vi "RH_BF_LD-400_MFLI_PK_v4.0_measure_voltageR_fourMFLI.vi"() -> ()   [LabVIEW 2016]
uses:
  <instrlib>/Zurich Instruments LabOne/Public/Configure/ziGetValueDemodSampleEx.vi
  <vilib>/Utility/file.llb/Write To Spreadsheet File (DBL).vi
  <instrlib>/Zurich Instruments LabOne/Zurich Instruments LabOne.lvlib
panel:
  in  "Magnet IP Address":string="169.254.50.121"
  in  "Current 4 (A)":dbl
  in  "Current 3 (A)":dbl
  in  "Current 2 (A)":dbl
  in  "Current 1 (A)":dbl
  in  "MFLI 4 Address":string="DEV3647"
  in  "Device 4 details:":string="ZrTe5_Rxy_24-32_10uA_7.919Hz"
  in  "Delay(s) after each data point":dbl=8.0 format="%#_13g"
  in  "Device 3 details:":string="ZrTe5_Rxx_35-32_10uA_7.919Hz"
  in  "MFLI 3 Address":string="DEV3647"
  in  "MFLI 2 Address":string="DEV4496"
  in  "MFLI 1 Address":string="DEV4382"
  in  "Device 2 details:":string="ZrTe5_Rxx_39-24_10uA_7.919Hz"
  in  "Device 1 details:":string="ZrTe5_Rxy_39-35_10uA_7.919Hz"
  in  "STOP":bool
  out "Device details":string="Device details: \rDevice 1 details: AJ0267-Ta3Sb(21nm)/TaN(2nm)/Sapphire (RT growth)\tDevice 1 details: AJ0268-Ta3Sb(21nm)/TaN(2nm)/Sapphire (1000C growth)\r\t"
  out "data":ext[](array[numeric])=[0.0080852, 9923.583, 0.16276936015514457, 1.6064700025522405e-08, 9.869609372556507e-08, 0.27307549143227666, 2.7272832558602143e-08, 9.987286817852663e-08]
  out "path":path=path "D:/Pranava/Data/Ta3Sb/15-07-2020/001_AJ0267+AJ0268_RT_cooldown_100nA"
  in  "Path":path=path "D:/Pranava/Data/Stan/12-06-2021/002_ZrTe5_RH_baseT"
  in  "Tab Control":enum32{"Page 1", "Page 2"}(tab)
  out "Resistance vs time":cluster{dbl[], dbl[]}[](graph)
  out "Resistance 1 (ohm)":dbl=0.16276936015514457 format="%#_13g"
  out "Voltage 1 (V)":dbl=1.6064700025522405e-08 format="%#_4g"
  out "elapsed time (min)":dbl=165.39305000000002
  out "elapsed time (s)":dbl=9923.583
  out "Magnetic Field (T)":dbl=0.0080852
  out "Resistance vs T":cluster{dbl[], dbl[]}[](graph)
  out "Voltage 2 (V)":dbl=2.7272832558602143e-08 format="%#_4g"
  out "Resistance 2 (ohm)":dbl=0.27307549143227666 format="%#_13g"
  out "Resistance 3 (ohm)":dbl format="%#_13g"
  out "Voltage 3 (V)":dbl=2.7272832558602143e-08 format="%#_4g"
  out "Resistance 4 (ohm)":dbl=0.16276936015514457 format="%#_13g"
  out "Voltage 4 (V)":dbl=2.7272832558602143e-08 format="%#_4g"
  out "Updates":string="- Using shift register to get data from MFLI\n- Using read demod instead of poll function\n- Measuring 4 devices using MFLI at the same time"
  out "Error Out":errorcluster
  # "Use this button to abort the measurement"
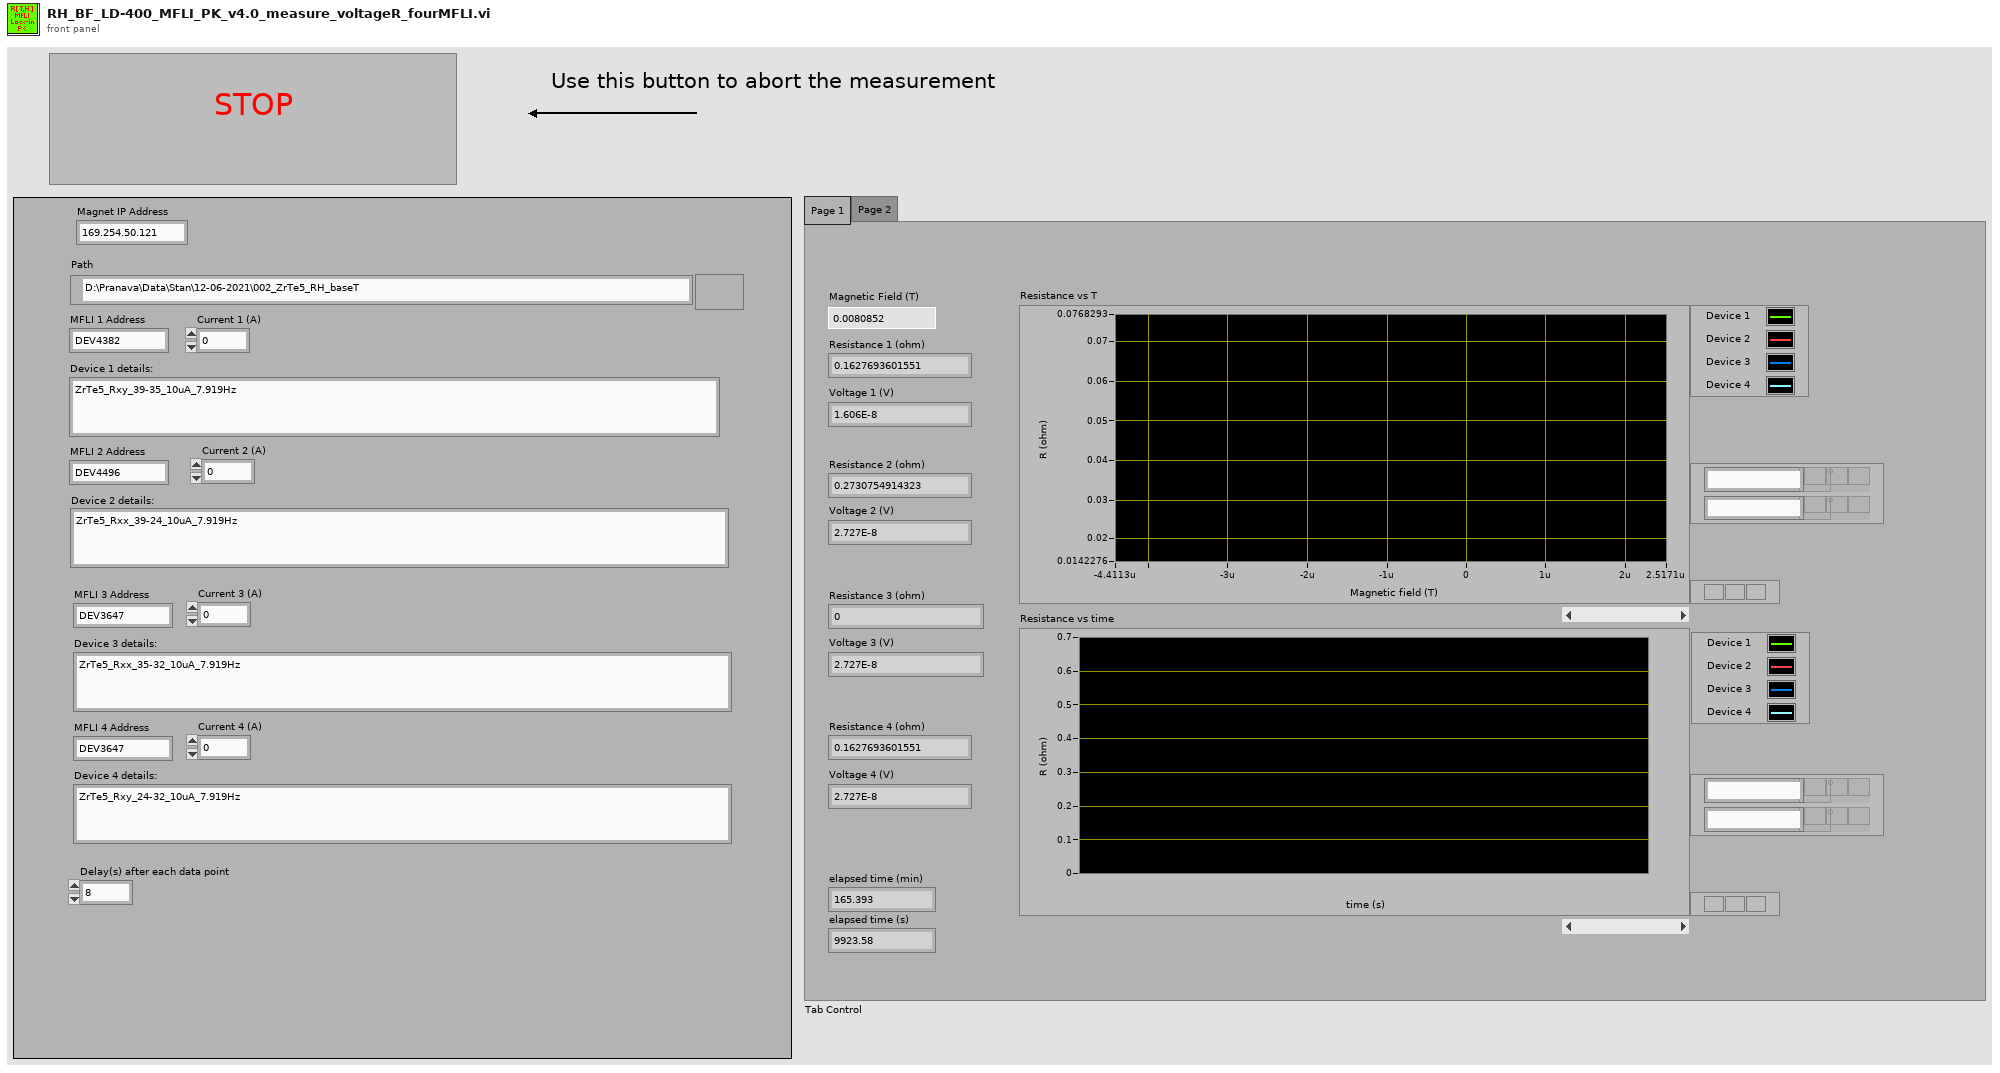
[diagram p1: front panel]
types:
  T1 = enum16{"open", "replace", "create", "open or create", "replace or create", "replace or create with confirmation"}
  T2 = typedef "Zurich Instruments LabOne.lvlib/ziTypeHandle.ctl" = cluster{"handleValid":bool, "Conn":u64, "Path Prefix":string, "Handle":u64, "Connected":bool, "Clockbase(s)":dbl}
  T3 = typedef "Zurich Instruments LabOne.lvlib/ziTypeDemodSampleSingle.ctl" = cluster{"Timestamps (ticks)":u64, "X (Vrms)":dbl, "Y (Vrms)":dbl, "Osc Phase (deg)":dbl, "Freq (Hz)":dbl, "DIO":u32, "AuxIn0 (V)":dbl, "AuxIn1 (V)":dbl, "Trigger":u32}
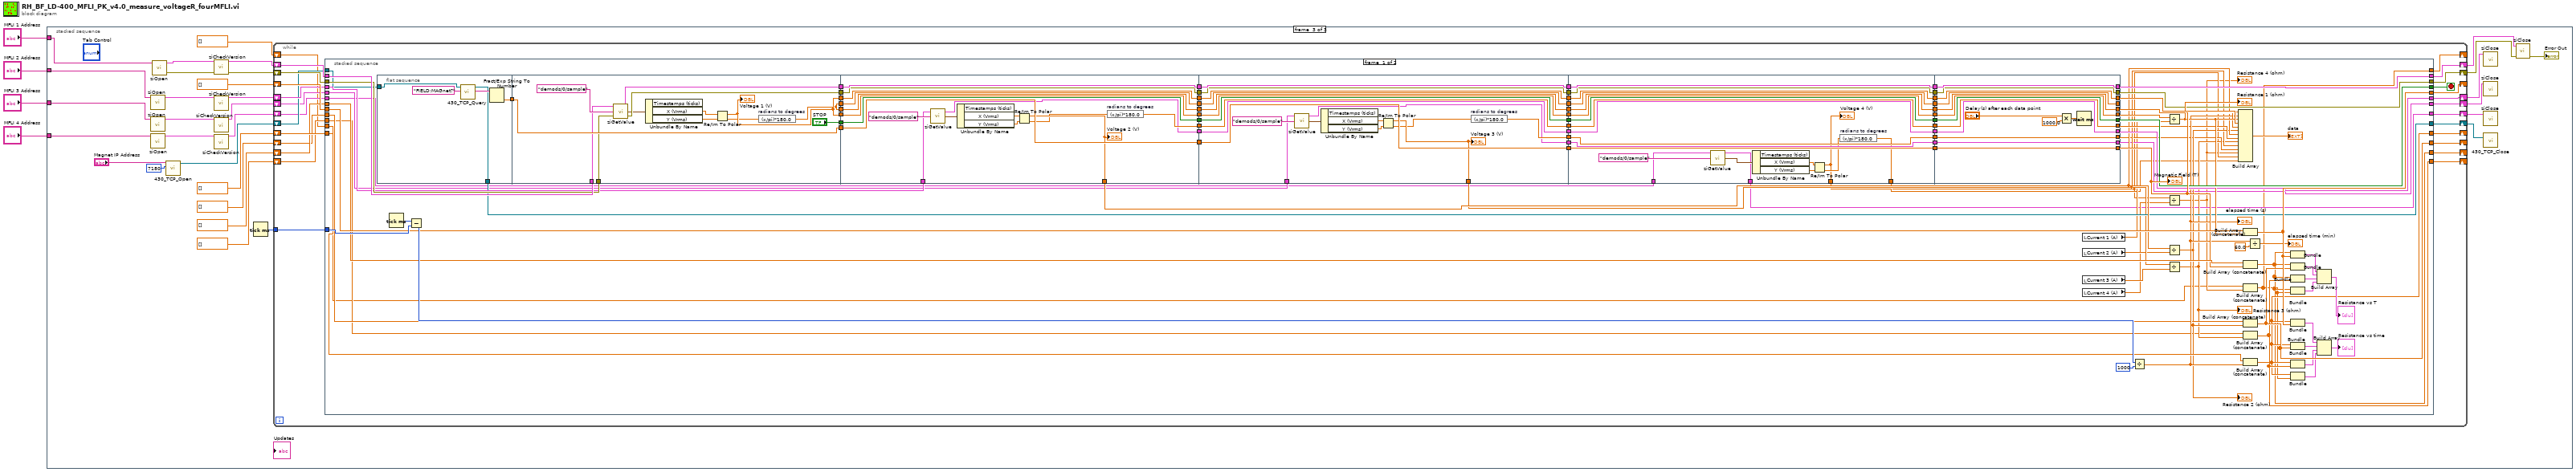
[diagram p0: block diagram]
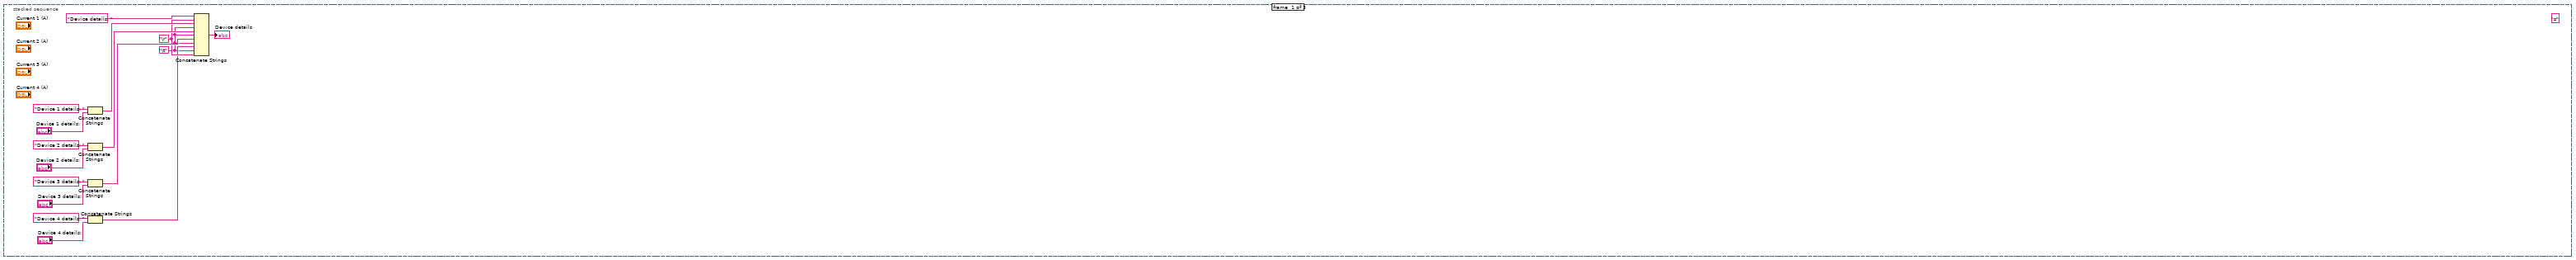
[diagram p2: hidden frame]
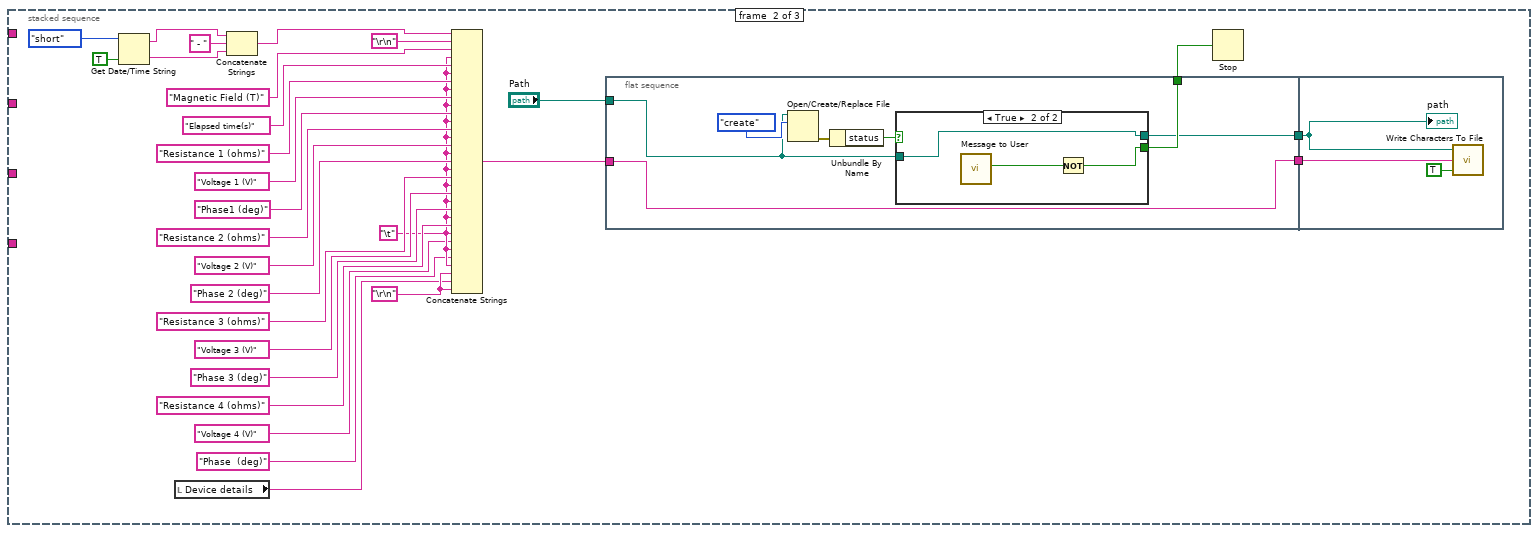
[diagram p3: hidden frame]
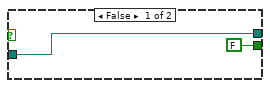
[diagram p4: hidden frame]
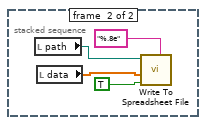
[diagram p5: hidden frame]
diagram:
  n1 = stacked-sequence {
    tunnel: "MFLI 1 Address" -> [_ _ w84]
    tunnel: "MFLI 2 Address" -> [_ _ w82]
    tunnel: "MFLI 3 Address" -> [_ _ w78]
    tunnel: "MFLI 4 Address" -> [_ _ w72]
    frame #0 {
      (unwired) "s"
      w7 = "\r"
      w5 = "\t"
      n2 = Concatenate Strings("Device 1 details: ", "Device 1 details:") -> (w14:string)
      n3 = Concatenate Strings("Device 2 details: ", "Device 2 details:") -> (w13:string)
      n4 = Concatenate Strings("Device 3 details: ", "Device 3 details:") -> (w10:string)
      n5 = Concatenate Strings("Device 4 details: ", "Device 4 details:") -> (w6:string)
      n6 = Concatenate Strings("Device details: ", w7, w14, w5, w13, w5, w10, w5, w6, w5, w7) -> (→"Device details":string)
    }
    frame #1 {
      w26 = "\r\n"
      w23 = "\t"
      n7 = Get Date/Time String(date format (0)=enum16{"short", "long", "abbreviated"}."short", want seconds? (F)=TRUE) -> (date string=w43:string, time string=w42:string)  [unwired: 1 in]
      n8 = local read "Device details"() -> (w25:string)
      n9 = Concatenate Strings(w43, " - " ("string"), w42) -> (w38:string)
      n10 = Concatenate Strings(w38, "\r\n", "Magnetic Field (T)" ("string"), w23, "Elapsed time(s)" ("string"), w23, "Resistance 1 (ohms)" ("string"), w23, "Voltage 1 (V)", w23, "Phase1 (deg)", w23, "Resistance 2 (ohms)" ("string"), w23, "Voltage 2 (V)", w23, "Phase 2 (deg)", w23, "Resistance 3 (ohms)" ("string"), w23, "Voltage 3 (V)", w23, "Phase 3 (deg)", w23, "Resistance 4 (ohms)" ("string"), w23, "Voltage 4 (V)", w23, "Phase  (deg)", w23, w26, w25, w26) -> (w47:string)
      n11 = flat-sequence {
        tunnel: "Path" -> [w50]
        tunnel: w47 -> [w53]
        tunnel: [w53] -> w46
        tunnel: [w52] -> w36
        tunnel: [w51] -> w39
        tunnel: w46 -> [w63]
        tunnel: w39 -> [w62]
        frame #0 {
          n12 = Open/Create/Replace File(file path (use dialog)=w50, operation (0:open)=T1."create") -> (error out=w56:errorcluster)  [unwired: 4 in, 2 out]
          n13 = Unbundle By Name(w56) -> ("status"=w54:bool)
          n14 = case shown="True" w54 {
            tunnel: [FALSE ("Yes") w60] -> w52
            tunnel: [w57 w59] -> w51
            tunnel: w50 -> [w57 w59]
            frame False {
            }
            frame True {
              n15 = call "Message to User"() -> ("Yes"=w61:bool)  [unwired: 10 in, 1 out]
              n16 = Not(x=w61) -> (.not. x?=w60:bool)
            }
          }
        }
        frame #1 {
          n17 = call <vilib>:"Write Characters To File.vi"("append to file? (new file:F)"=TRUE, "character string"=w63, "file path (dialog if empty)"=w62) -> ()  [unwired: 2 in, 1 out]
          "path" <- w62
        }
      }
      n18 = Stop(stop? (T)=w36) -> ()
    }
    frame #2 {
      n19 = call <instrlib>:"ziOpen.vi"("Address"=w82) -> ("HandleOut"=w83:T2)  [unwired: 3 in, 2 out]
      n20 = call <instrlib>:"ziOpen.vi"("Address"=w78) -> ("HandleOut"=w77:T2)  [unwired: 3 in, 2 out]
      n21 = call <instrlib>:"ziOpen.vi"("Address"=w72) -> ("HandleOut"=w73:T2)  [unwired: 3 in, 2 out]
      n22 = call <instrlib>:"ziOpen.vi"("Address"=w84) -> ("Error Out"=w90:errorcluster, "HandleOut"=w91:T2)  [unwired: 3 in, 1 out]
      n23 = call "430_TCP_Open.vi"("IP Address"="Magnet IP Address", "TCP Port"=7180) -> ("connection ID"=w66:refnum<k5>)  [unwired: 4 in, 2 out]
      n24 = call <instrlib>:"ziCheckVersion.vi"("Handle In"=w91, "Error In"=w90) -> ("Handle Out"=w89:T2, "Error Out"=w86:errorcluster)  [unwired: 11 in, 1 out]
      n25 = call <instrlib>:"ziCheckVersion.vi"("Handle In"=w83) -> ("Handle Out"=w80:T2)  [unwired: 12 in, 2 out]
      n26 = call <instrlib>:"ziCheckVersion.vi"("Handle In"=w77) -> ("Handle Out"=w76:T2)  [unwired: 12 in, 2 out]
      n27 = call <instrlib>:"ziCheckVersion.vi"("Handle In"=w73) -> ("Handle Out"=w70:T2)  [unwired: 12 in, 2 out]
      n28 = Tick Count (ms)() -> (millisecond timer value=w94:u32)
      n29 = while {
        shift-right: [w116] -> _
        shift-left: dbl[] [] -> [w121]
        tunnel: w94 -> [w120]
        shift-right: [w115] -> _
        shift-left: dbl[] [] -> [w119]
        shift-right: [w117] -> _
        shift-left: dbl[] [] -> [w118]
        shift-right: [w112] -> w88
        shift-left: w89 -> [w114]
        shift-right: [w110] -> w85
        shift-left: w86 -> [w111]
        shift-right: [w109] -> w81
        shift-left: w80 -> [w108]
        shift-right: [w106] -> _
        shift-left: dbl[] [] -> [w107]
        shift-right: [w104] -> w65
        shift-left: w66 -> [w105]
        shift-right: [w102] -> w75
        shift-left: w76 -> [w103]
        shift-right: [w100] -> _
        shift-left: dbl[] [] -> [w101]
        shift-right: [w99] -> w71
        shift-left: w70 -> [w98]
        shift-right: [w96] -> _
        shift-left: dbl[] [] -> [w97]
        stop <- w113 stop-if-true
        n30 = stacked-sequence {
          tunnel: w121 -> [w221 _]
          tunnel: w120 -> [w225 _]
          tunnel: w119 -> [w222 _]
          tunnel: w118 -> [w220 _]
          tunnel: [w124 _] -> w117
          tunnel: [w219 _] -> w116
          tunnel: [w126 _] -> w115
          tunnel: [w212 _] -> w113
          tunnel: w114 -> [w208 _]
          tunnel: [w207 _] -> w112
          tunnel: w111 -> [w206 _]
          tunnel: [w205 _] -> w110
          tunnel: w108 -> [w195 _]
          tunnel: [w194 _] -> w109
          tunnel: w107 -> [w190 _]
          tunnel: [w185 _] -> w106
          tunnel: w105 -> [w181 _]
          tunnel: [w180 _] -> w104
          tunnel: w103 -> [w169 _]
          tunnel: [w166 _] -> w102
          tunnel: w101 -> [w162 _]
          tunnel: [w161 _] -> w100
          tunnel: w98 -> [w130 _]
          tunnel: [w129 _] -> w99
          tunnel: w97 -> [w123 _]
          tunnel: [w122 _] -> w96
          frame #0 {
            n31 = flat-sequence {
              tunnel: w181 -> [w228]
              tunnel: [w227] -> w204
              tunnel: [w226] -> w180
              tunnel: [w243] -> w203
              tunnel: [w242] -> w202
              tunnel: ["STOP"] -> w201
              tunnel: [w243] -> w200
              tunnel: [w240] -> w199
              tunnel: [w240] -> w198
              tunnel: [w239] -> w197
              tunnel: [w238] -> w196
              tunnel: w206 -> [w234]
              tunnel: w208 -> [w235]
              tunnel: w204 -> [w242]
              tunnel: [w260] -> w179
              tunnel: [w259] -> w178
              tunnel: [w258] -> w177
              tunnel: [w257] -> w176
              tunnel: [w256] -> w175
              tunnel: [w255] -> w174
              tunnel: [w254] -> w173
              tunnel: [w253] -> w172
              tunnel: [w251] -> w171
              tunnel: [w252] -> w170
              tunnel: [w245] -> w191
              tunnel: w195 -> [w249]
              tunnel: w196 -> [w253]
              tunnel: w197 -> [w254]
              tunnel: w198 -> [w255]
              tunnel: w199 -> [w256]
              tunnel: w200 -> [w257]
              tunnel: w201 -> [w258]
              tunnel: w202 -> [w259]
              tunnel: w203 -> [w260]
              tunnel: [w279] -> w156
              tunnel: [w278] -> w154
              tunnel: [w277] -> w152
              tunnel: [w276] -> w150
              tunnel: [w275] -> w148
              tunnel: [w274] -> w146
              tunnel: [w273] -> w144
              tunnel: [w272] -> w142
              tunnel: [w271] -> w140
              tunnel: [w270] -> w138
              tunnel: [w269] -> w136
              tunnel: [w268] -> w134
              tunnel: [w262] -> w168
              tunnel: w169 -> [w263]
              tunnel: w170 -> [w270]
              tunnel: w171 -> [w271]
              tunnel: w172 -> [w272]
              tunnel: w173 -> [w273]
              tunnel: w174 -> [w274]
              tunnel: w175 -> [w275]
              tunnel: w176 -> [w276]
              tunnel: w177 -> [w277]
              tunnel: w178 -> [w278]
              tunnel: w179 -> [w279]
              tunnel: w156 -> [w300]
              tunnel: [w300] -> w155
              tunnel: w154 -> [w299]
              tunnel: [w299] -> w153
              tunnel: w152 -> [w298]
              tunnel: [w298] -> w151
              tunnel: w150 -> [w297]
              tunnel: [w297] -> w149
              tunnel: w148 -> [w296]
              tunnel: [w296] -> w147
              tunnel: w146 -> [w295]
              tunnel: [w295] -> w145
              tunnel: w144 -> [w294]
              tunnel: [w294] -> w143
              tunnel: w142 -> [w293]
              tunnel: [w293] -> w141
              tunnel: w140 -> [w292]
              tunnel: [w292] -> w139
              tunnel: w138 -> [w291]
              tunnel: [w291] -> w137
              tunnel: w136 -> [w290]
              tunnel: [w290] -> w135
              tunnel: w134 -> [w289]
              tunnel: [w289] -> w133
              tunnel: [w283] -> w131
              tunnel: [w282] -> w132
              tunnel: w130 -> [w281]
              tunnel: [w280] -> w129
              tunnel: [w304] -> w166
              tunnel: [w305] -> w167
              tunnel: [w306] -> w192
              tunnel: [w307] -> w194
              tunnel: [w308] -> w205
              tunnel: [w309] -> w207
              tunnel: [w310] -> w209
              tunnel: [w311] -> _
              tunnel: [w312] -> w211
              tunnel: [w313] -> w212
              tunnel: [w314] -> w213
              tunnel: [w315] -> w215
              tunnel: w155 -> [w315]
              tunnel: w153 -> [w314]
              tunnel: w151 -> [w313]
              tunnel: w149 -> [w312]
              tunnel: w147 -> [w311]
              tunnel: w145 -> [w310]
              tunnel: w143 -> [w309]
              tunnel: w141 -> [w308]
              tunnel: w139 -> [w307]
              tunnel: w137 -> [w306]
              tunnel: w135 -> [w305]
              tunnel: w133 -> [w304]
              frame #0 {
                n32 = call "430_TCP_Query.vi"("Command"="FIELD:MAGnet?", "connection ID"=w228) -> ("Response"=w229:string, "connection ID out"=w226:refnum<k5>)  [unwired: 5 in, 3 out]
                n33 = Fract/Exp String To Number(string=w229) -> (number=w227:dbl)  [unwired: 3 in, 1 out]
              }
              frame #1 {
                n34 = call-poly <instrlib>:"ziGetValue.vi"("error in"=w234, "Path"="demods/0/sample", "Handle In"=w235) -> ("error out"=w238:errorcluster, "Demod Sample Out"=w236:T3, "Handle Out"=w239:T2)
                n35 = Unbundle By Name(w236) -> ("X (Vrms)"=w233:dbl, "Y (Vrms)"=w232:dbl)  [unwired: 1 out]
                n36 = Re/Im To Polar(2:w232, 3:w233) -> (0:w231:dbl, 1:w243:dbl)
                "Voltage 1 (V)" <- w243
                n37 = expression code="(x/pi)*180.0" "radians to degrees"(w231) -> (w240:dbl)
              }
              frame #2 {
                n38 = call-poly <instrlib>:"ziGetValue.vi"("Path"="demods/0/sample", "Handle In"=w249) -> ("Demod Sample Out"=w248:T3, "Handle Out"=w251:T2)  [unwired: 1 in, 1 out]
                n39 = Unbundle By Name(w248) -> ("X (Vrms)"=w247:dbl, "Y (Vrms)"=w246:dbl)  [unwired: 1 out]
                n40 = Re/Im To Polar(2:w246, 3:w247) -> (0:w244:dbl, 1:w245:dbl)
                "Voltage 2 (V)" <- w245
                n41 = expression code="(x/pi)*180.0" "radians to degrees"(w244) -> (w252:dbl)
              }
              frame #3 {
                n42 = call-poly <instrlib>:"ziGetValue.vi"("Path"="demods/0/sample", "Handle In"=w263) -> ("Demod Sample Out"=w266:T3, "Handle Out"=w268:T2)  [unwired: 1 in, 1 out]
                n43 = Unbundle By Name(w266) -> ("X (Vrms)"=w265:dbl, "Y (Vrms)"=w264:dbl)  [unwired: 1 out]
                n44 = Re/Im To Polar(2:w264, 3:w265) -> (0:w261:dbl, 1:w262:dbl)
                "Voltage 3 (V)" <- w262
                n45 = expression code="(x/pi)*180.0" "radians to degrees"(w261) -> (w269:dbl)
              }
              frame #4 {
                n46 = call-poly <instrlib>:"ziGetValue.vi"("Path"="demods/0/sample", "Handle In"=w281) -> ("Demod Sample Out"=w285:T3, "Handle Out"=w280:T2)  [unwired: 1 in, 1 out]
                n47 = Unbundle By Name(w285) -> ("X (Vrms)"=w287:dbl, "Y (Vrms)"=w286:dbl)  [unwired: 1 out]
                n48 = Re/Im To Polar(2:w286, 3:w287) -> (0:w284:dbl, 1:w283:dbl)
                "Voltage 4 (V)" <- w283
                n49 = expression code="(x/pi)*180.0" "radians to degrees"(w284) -> (w282:dbl)
              }
              frame #5 {
                n50 = Multiply(x="Delay(s) after each data point", y=1000.0) -> (x*y=w303:dbl)
                n51 = Wait (ms)(milliseconds to wait=w303) -> ()  [unwired: 1 out]
              }
            }
            n52 = Tick Count (ms)() -> (millisecond timer value=w223:u32)
            n53 = Subtract(x=w223, y=w225) -> (x-y=w224:u32)
            n54 = local read "Current 1 (A)"() -> (w160:dbl)
            n55 = local read "Current 2 (A)"() -> (w159:dbl)
            n56 = local read "Current 3 (A)"() -> (w158:dbl)
            n57 = local read "Current 4 (A)"() -> (w157:dbl)
            n58 = Divide(x=w224, y=u32 1000) -> (x/y=w193:dbl)
            "elapsed time (s)" <- w193
            n59 = Divide(x=w211, y=w160) -> (x/y=w210:dbl)
            "Resistance 1 (ohm)" <- w210
            n60 = Divide(x=w131, y=w157) -> (x/y=w127:dbl)
            "Resistance 4 (ohm)" <- w127
            n61 = Divide(x=w191, y=w159) -> (x/y=w189:dbl)
            "Resistance 2 (ohm)" <- w189
            n62 = Divide(x=w168, y=w158) -> (x/y=w165:dbl)
            "Resistance 3 (ohm)" <- w165
            n63 = Build Array(w213, w193, w210, w215, w209, w189, w191, w192, w165, w168, w167, w127, w131, w132) -> (→"data":dbl[])
            n64 = Build Array (concatenate)(w221, w210) -> (w219:dbl[])
            n65 = Build Array (concatenate)(w123, w127) -> (w122:dbl[])
            n66 = Build Array (concatenate)(w190, w189) -> (w185:dbl[])
            n67 = Build Array (concatenate)(w162, w165) -> (w161:dbl[])
            n68 = Build Array (concatenate)(w220, w213) -> (w124:dbl[])
            n69 = Build Array (concatenate)(w222, w193) -> (w126:dbl[])
            n70 = Divide(x=w193, y=60.0) -> (x/y=→"elapsed time (min)":dbl)
            n71 = Bundle(w124, w219) -> (w183:cluster{dbl[], dbl[]})  [unwired: 1 in]
            n72 = Bundle(w124, w185) -> (w184:cluster{dbl[], dbl[]})  [unwired: 1 in]
            n73 = Bundle(w124, w161) -> (w164:cluster{dbl[], dbl[]})  [unwired: 1 in]
            n74 = Bundle(w124, w122) -> (w125:cluster{dbl[], dbl[]})  [unwired: 1 in]
            n75 = Bundle(w126, w219) -> (w188:cluster{dbl[], dbl[]})  [unwired: 1 in]
            n76 = Bundle(w126, w185) -> (w187:cluster{dbl[], dbl[]})  [unwired: 1 in]
            n77 = Bundle(w126, w161) -> (w163:cluster{dbl[], dbl[]})  [unwired: 1 in]
            n78 = Bundle(w126, w122) -> (w128:cluster{dbl[], dbl[]})  [unwired: 1 in]
            n79 = Build Array(w183, w184, w164, w125) -> (→"Resistance vs T":cluster{dbl[], dbl[]}[])
            n80 = Build Array(w188, w187, w163, w128) -> (→"Resistance vs time":cluster{dbl[], dbl[]}[])
            "Magnetic Field (T)" <- w213
          }
          frame #1 {
            n81 = local read "path"() -> (w319:path)
            n82 = local read "data"() -> (w317:ext[])
            n83 = call-poly <vilib>:"Write To Spreadsheet File.vi"("format (%.3f)"="%.8e", "append to file? (new file:F)"=TRUE, "1D data"=w317, "file path (dialog if empty)"=w319) -> ()  [unwired: 4 in, 1 out]
          }
        }
      }
      n84 = call <instrlib>:"ziClose.vi"("Handle In"=w81) -> ()  [unwired: 1 in, 4 out]
      n85 = call <instrlib>:"ziClose.vi"("Handle In"=w75) -> ()  [unwired: 1 in, 4 out]
      n86 = call <instrlib>:"ziClose.vi"("Handle In"=w71) -> ()  [unwired: 1 in, 4 out]
      n87 = call "430_TCP_Close.vi"("connection ID"=w65) -> ()  [unwired: 1 in, 2 out]
      n88 = call <instrlib>:"ziClose.vi"("Error In"=w85, "Handle In"=w88) -> ("Error Out"=→"Error Out":errorcluster)  [unwired: 3 out]
    }
  }
